vi "Run Filter.vi"(8 "error in (no error)":errorcluster, 10 "resource entries in":T1(array[cluster]) {"FPGA CD Ref" format="%.0x"; "reserver" format="%.0x"}, 11 "RIO Device Filter in":refnum<class "RIO Device Filter.lvclass">) -> (0 "error out":errorcluster, 2 "resource entries out":T1(array[cluster]) {"FPGA CD Ref" format="%.0x"; "reserver" format="%.0x"})   [LabVIEW 2016, in "RIO Device Filter.lvclass"]
uses:
  FPGA RM Test Client Configuration.llb/RIO Device Filter.lvclass
  FPGA RM Test Client Configuration.llb/RIO Device Filter.lvclass/RIO Device Filter.ctl
  FPGA RM Test Client Configuration.llb/Constants.vi
  FPGA RM Test Client Configuration.llb/FPGA Addon Shared.lvlib
  FPGA RM Test Client Configuration.llb/Custom Device API.lvlib
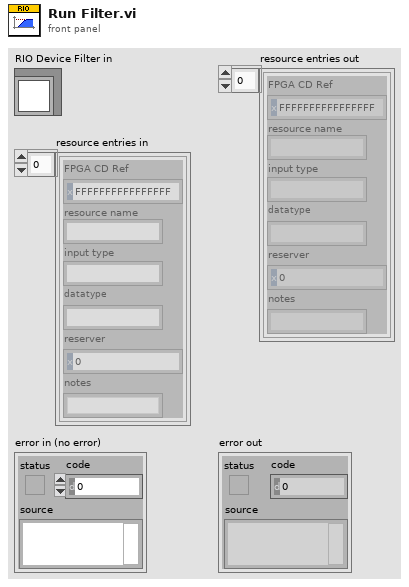
[diagram p1: front panel]
types:
  T1 = cluster{"FPGA CD Ref":u64, "resource name":string, "input type":string, "datatype":string, "reserver":u64, "notes":string}[]
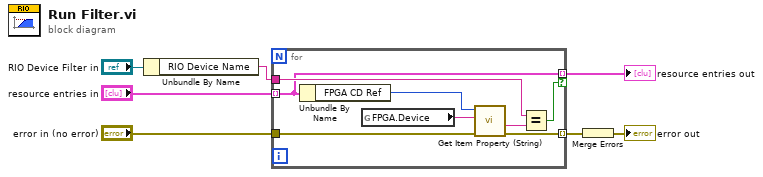
[diagram p0: block diagram]
diagram:
  n1 = Unbundle By Name("RIO Device Filter in") -> ("RIO Device Name"=w5:string)
  n2 = for {
    tunnel: "resource entries in" -> [w11] mode=indexing
    tunnel: w5 -> [w12]
    tunnel: [w11] -> w4 mode=indexing if=w10
    tunnel: "error in (no error)" -> [w9]
    tunnel: [w8] -> w2 mode=indexing
    n3 = Unbundle By Name(w11) -> ("FPGA CD Ref"=w14:u64)
    n4 = global read "Constants.vi" "FPGA.Device"() -> (w15:string)
    n5 = call "Get Item Property (String).vi"("error in (no error)"=w9, "Property Name"=w15, "Item Ref in"=w14) -> ("error out"=w8:errorcluster, "Value"=w13:string)  [unwired: 5 in, 2 out]
    n6 = Equal?(x=w12, y=w13) -> (x = y?=w10:bool)
  }
  "resource entries out" <- w4
  n7 = Merge Errors(w2) -> (→"error out":errorcluster)
